vi "(Signed) Index 1D Array [String].vi"(8 "Signed Index":i32, 10 "Array":string[](array[string])) -> (0 "Out of Range?":bool, 2 "Array Element":string)   [LabVIEW 2019]
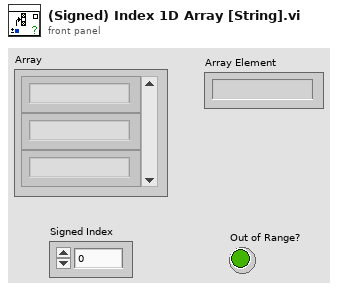
[diagram p1: front panel]
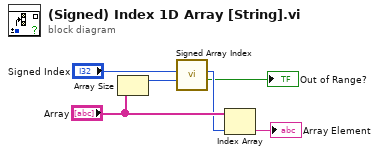
[diagram p0: block diagram]
diagram:
  n1 = Array Size(array="Array") -> (size(s)=w5:i32)
  n2 = call "Signed Array Index.vi"("Array Size"=w5, "Array Index in"="Signed Index") -> ("Out of Range?"=→"Out of Range?":bool, "Array Index out"=w3:i32)  [unwired: 8 in]
  n3 = Index Array(array="Array", index=w3) -> (element=→"Array Element":string)
